vi "S8300E_Revision_Test_WIH.vi"() -> ()   [LabVIEW 2011]
panel:
  out "PRELOG2":string
  out "PRELOG1":string
  out "UUT_LAN_FW_VERSION":string
  out "CPK_SUFFIX":string
  out "Vintage_Number":string
  out "CPLD_Version":string
  out "Log":string
  out "MSG List":string[](array[string])
  out "VISA resource name out":refnum<visa-resource-name>
  out "Cmd Line":cluster{string, string, "BIST Version":string}[](array[cluster])
  out "BIST Version":string
  out "OS Version":string
  out "BIOS_VERSION":string
  out "BEGIN TIME":u32
  out "進行狀況":string
  # "Error Code:Version\nError Code:UART"
  # "2015-6-1"
  # "S8300E Version Check (接UART COM9)"
  # "Baud-Rate:115200"
  # "Step1:BIOS Version Check\nStep2:OS Version\nStep3:BIST\nStep4:Get CPLD device ID and revision number\nStep5:Get Vintage Number of the Circuit Pack\nStep6:Get Suffix of the Circuit Pack\nStep7:Get SuperIO Device ID\nStep8:Get Clock Generator ID\nStep9:Get LAN EEPROM firmware verson"
  # "Rule :bits [7-4] : CPLD Device ID, S8300E CPLD Device ID=4\nbits [3-0] : CPLD Revision Number"
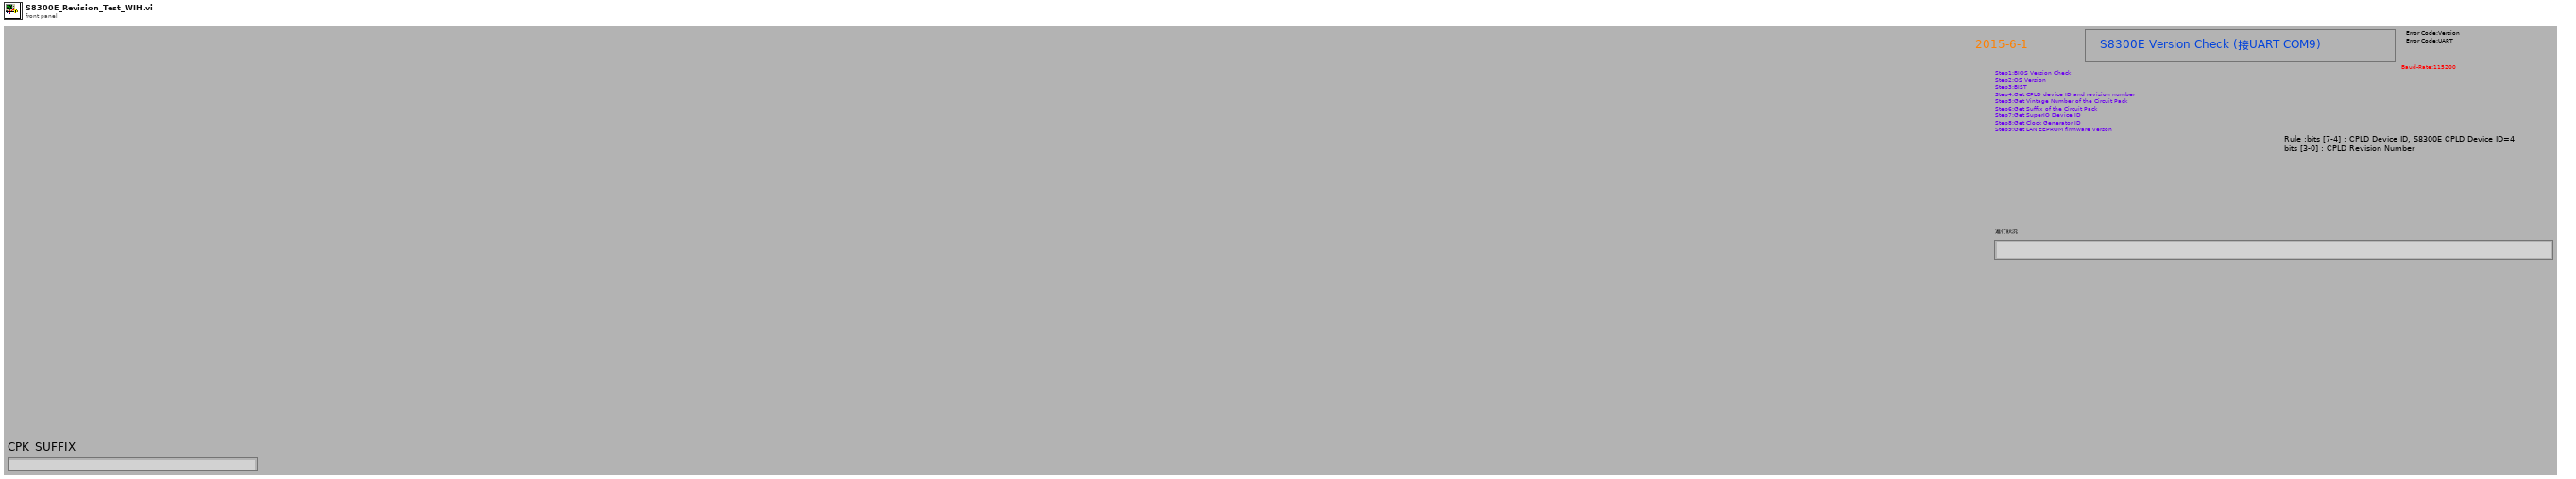
[diagram p1: front panel]
types:
  T1 = cluster{string, string, "UUT_LAN_FW_VERSION":string}
  T2 = cluster{string, string, "UUT_LAN_FW_VERSION":string}[]
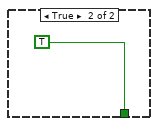
[diagram p5: hidden frame]
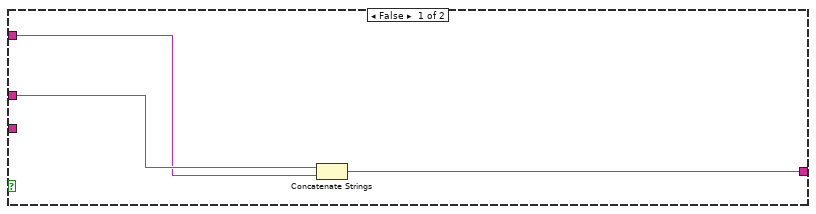
[diagram p6: hidden frame]
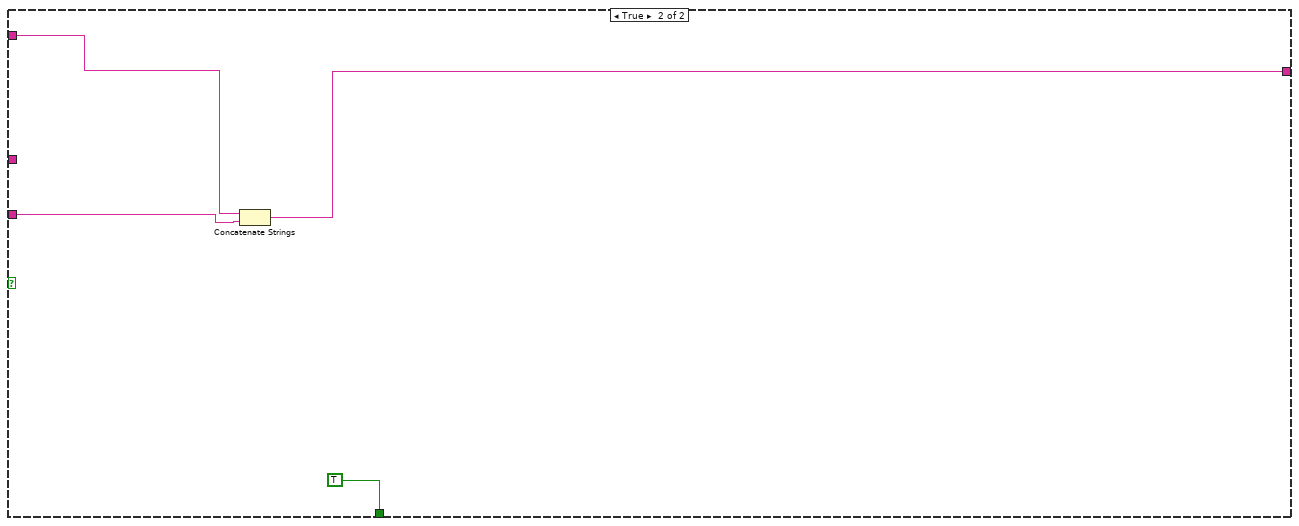
[diagram p7: hidden frame]
diagram:
  n1 = flat-sequence {
    frame #0 {
      n2 = Tick Count (ms)() -> (millisecond timer value=→"BEGIN TIME":u32)
    }
    frame #1 {
      n3 = property on="進行狀況" class="Str"("Blinking"=TRUE) -> ()  [unwired: 2 in, 2 out]
      "進行狀況" <- "進入測試準備中...." ("進行狀況")
    }
    frame #2 {
      n4 = call "SUB_SearchFile_inFolder.vi"("Search Filename in Folder"="S8300E_sfcs_misc.txt") -> ("File Existing True/Flase"=w4:bool)  [unwired: 1 in]
      n5 = case shown="False" w4 {
        frame False {
          n6 = flat-sequence {
            frame #0 {
              n7 = call "Display Message to User"() -> ()  [unwired: 10 in, 2 out]
            }
            frame #1 {
              n8 = call "SUB_Writelog.vi"("Pass/Fail"="Fail:S8300E_Revision_Test") -> ()  [unwired: 2 in]
            }
            frame #2 {
              n9 = Quit LabVIEW(quit? (T)=TRUE) -> ()
            }
          }
        }
        frame True {
        }
      }
    }
    frame #3 {
      n10 = call "SUB_ReadScript_File.vi"("Script FileName"="S8300E_sfcs_misc.txt" ("Search Filename in Folder")) -> ("text"=w12:string)  [unwired: 1 in, 2 out]
      n11 = call "SUB_FindSpecificString.vi"("Find this String"="UUT_CPLD_VERSION=", "String data"=w12) -> ("before \"; \" string"=→"CPLD_Version":string, "Found"=w17:bool)  [unwired: 2 in]
      n12 = call "SUB_FindSpecificString.vi"("Find this String"="UUT_OS_VERSION=", "String data"=w12) -> ("before \"; \" string"=→"OS Version":string, "Found"=w28:bool)  [unwired: 2 in]
      n13 = call "SUB_FindSpecificString.vi"("Find this String"="UUT_BIST_VERSION=", "String data"=w12) -> ("before \"; \" string"=→"BIST Version":string, "Found"=w26:bool)  [unwired: 2 in]
      n14 = call "SUB_FindSpecificString.vi"("Find this String"="UUT_VintageNumber=", "String data"=w12) -> ("before \"; \" string"=→"Vintage_Number":string, "Found"=w19:bool)  [unwired: 2 in]
      n15 = call "SUB_FindSpecificString.vi"("Find this String"="UUT_CircuitPack_SUFFIX=", "String data"=w12) -> ("before \"; \" string"=→"CPK_SUFFIX":string, "Found"=w18:bool)  [unwired: 2 in]
      n16 = call "SUB_FindSpecificString.vi"("Find this String"="UUT_BIOS_VERSION=", "String data"=w12) -> ("before \"; \" string"=→"BIOS_VERSION":string, "Found"=w29:bool)  [unwired: 2 in]
      n17 = call "SUB_FindSpecificString.vi"("Find this String"="UUT_LAN_FW_VERSION=", "String data"=w12) -> ("before \"; \" string"=→"UUT_LAN_FW_VERSION":string, "Found"=w10:bool)  [unwired: 2 in]
      n18 = And(x=w19, y=w18) -> (x .and. y?=w11:bool)
      n19 = And(x=w11, y=w10) -> (x .and. y?=w9:bool)
      n20 = And(x=w17, y=w9) -> (x .and. y?=w15:bool)
      n21 = And(x=w29, y=w28) -> (x .and. y?=w27:bool)
      n22 = And(x=w27, y=w26) -> (x .and. y?=w16:bool)
      n23 = And(x=w16, y=w15) -> (x .and. y?=w14:bool)
      n24 = case shown="False" w14 {
        frame False {
          n25 = flat-sequence {
            frame #0 {
              n26 = call "Display Message to User2"() -> ()  [unwired: 10 in, 2 out]
            }
            frame #1 {
              n27 = call "SUB_Writelog.vi"("Pass/Fail"="Fail:S8300E_Revision_Test") -> ()  [unwired: 2 in]
            }
            frame #2 {
              n28 = Quit LabVIEW(quit? (T)=TRUE) -> ()
            }
          }
        }
        frame True {
        }
      }
    }
    frame #4 {
      (unwired) "PASSED="
      (unwired) "PASSED="
      n29 = local read "BIST Version"() -> (w44:string)
      n30 = local read "OS Version"() -> (w48:string)
      n31 = local read "BIOS_VERSION"() -> (w53:string)
      n32 = local read "CPLD_Version"() -> (w83:string)
      n33 = local read "Vintage_Number"() -> (w80:string)
      n34 = local read "UUT_LAN_FW_VERSION"() -> (w40:string)
      n35 = local read "CPK_SUFFIX"() -> (w77:string)
      n36 = Concatenate Strings("PASSED=", w53, ";") -> (w51:string)
      n37 = Concatenate Strings("PASSED=", w48, ";") -> (w47:string)
      n38 = Concatenate Strings("PASSED=", w44, ";") -> (w43:string)
      n39 = Concatenate Strings("PASSED=", w40, ";") -> (w39:string)
      n40 = Bundle("./ver.sh -t", w43, "BIST Version"=w44) -> (w94:cluster{string, string, "BIST Version":string})  [unwired: 1 in]
      n41 = Bundle("./ver.sh -b", w51, "BIOS_VERSION"=w53) -> (w96:cluster{string, string, "BIOS_VERSION":string})  [unwired: 1 in]
      n42 = Bundle("./ver.sh -o", w47, "OS Version"=w48) -> (w95:cluster{string, string, "OS Version":string})  [unwired: 1 in]
      n43 = Bundle("./ver.sh -v", "PASSED=", "Vintage_Number"=w80) -> (w75:cluster{string, string, "Vintage_Number":string})  [unwired: 1 in]
      n44 = Bundle("./ver.sh -c", "PASSED=", "CPLD_Version"=w83) -> (w76:cluster{string, string, "CPLD_Version":string})  [unwired: 1 in]
      n45 = Bundle("./ver.sh -s", "PASSED=", "CPK_SUFFIX"=w77) -> (w74:cluster{string, string, "CPK_SUFFIX":string})  [unwired: 1 in]
      n46 = Bundle("./ver.sh -g", "PASSED=", "0X42") -> (w65:cluster{string, string, string})  [unwired: 1 in]
      n47 = Bundle("./eth.sh -f  1", w39, "UUT_LAN_FW_VERSION"=w40) -> (w60:T1)  [unwired: 1 in]
      n48 = Bundle("./eth.sh -f  2", w39, "UUT_LAN_FW_VERSION"=w40) -> (w59:T1)  [unwired: 1 in]
      n49 = Bundle("./ver.sh -p", "PASSED=", "Found IT8612F chip at 0xa20") -> (w70:cluster{string, string, string})  [unwired: 1 in]
      n50 = Bundle("./eth.sh -f   3", w39, "UUT_LAN_FW_VERSION"=w40) -> (w58:T1)  [unwired: 1 in]
      n51 = Build Array("正在處理BIOS版本中....", "正在處理OS版本中....", "正在處理BIST版本中....", "正在處理CPLD版本中....", "正在處理 Vintage Number of the Circuit Pack....", "正在處理Suffix of the Circuit Pack....", "正在處理SuperIO Device", "Get Clock Generator ID", "Get  LAN FW Version Port1", "Get  LAN FW Version Port2", "Get  LAN FW Version Port3") -> (→"MSG List":string[])
      n52 = Build Array(w96, w95, w94, w76, w75, w74, w70, w65, w60, w59, w58) -> (→"Cmd Line":T2)
    }
    frame #5 {
      n53 = call "SUB_COM1_CLOSE.vi"("VISA resource name"=refnum<visa-resource-name> "COM9") -> ()  [unwired: 3 in]
    }
    frame #6 {
      n54 = call "SUB_COM9_INIT.vi"("baud rate"=u32 115200) -> ("VISA resource name out"=w104:refnum<visa-resource-name>)  [unwired: 1 in, 1 out]
      "VISA resource name out" <- w104
      n55 = call "SUB_COM1Wrt.vi"("VISA resource name"=w104, "write buffer"="\r") -> ("duplicate VISA resource name"=w101:refnum<visa-resource-name>)  [unwired: 1 in, 1 out]
      n56 = call "SUB_ContinueCom1Read.vi"("Numeric"=1200, "duplicate VISA resource name 2"=w101) -> ()  [unwired: 1 in, 3 out]
    }
    frame #7 {
      n57 = while {
        stop <- w115 stop-if-true
        n58 = Tick Count (ms)() -> (millisecond timer value=w109:u32)
        n59 = local read "VISA resource name out"() -> (w107:refnum<visa-resource-name>)
        n60 = call "SUB_ContinueCom1Read.vi"("Numeric"=1200, "duplicate VISA resource name 2"=w107) -> ("duplicate VISA resource name"=w106:refnum<visa-resource-name>)  [unwired: 1 in, 2 out]
        n61 = call "SUB_COM1Wrt.vi"("VISA resource name"=w106, "write buffer"="\r") -> ("duplicate VISA resource name"=w111:refnum<visa-resource-name>)  [unwired: 1 in, 1 out]
        n62 = call "SUB_READ_COM1_FindString_timeout.vi"("Find this String"="S8300E", "Timeout Seccond"=2.0, "Begin time"=w109, "duplicate VISA resource name 2"=w111) -> ("Output String"=w112:string, "Found String"=w113:bool)  [unwired: 1 in, 1 out]
        n63 = case shown="False" w113 {
          tunnel: w112 -> [w121 _]
          tunnel: [w117 TRUE] -> w115
          frame False {
            n64 = call "SUB_YESNO.vi"("Debug View"=w121, "Status"="UART無正確反應!需有S8300E字串") -> ("yes/no"=w120:enum32{"No Selection", "Yes", "No", "None"})  [unwired: 1 in]
            n65 = Equal?(x=w120, y=enum32{"No Selection", "Yes", "No", "None"}."No") -> (x = y?=w118:bool)
            n66 = case shown="True" w118 {
              tunnel: [_ w123] -> w117
              frame False {
              }
              frame True {
                n67 = flat-sequence {
                  tunnel: [w127] -> w123
                  frame #0 {
                    n68 = call "SUB_Writelog.vi"("Pass/Fail"="Fail:S8300E_Revision_Test") -> ()  [unwired: 2 in]
                  }
                  frame #1 {
                    n69 = call "SUB_SFCS_SendResult.vi"("ErrorCode"="UART", "PASS_Fail (1/0)"=i8 0) -> ()  [unwired: 1 out]
                  }
                  frame #2 {
                    w127 = TRUE ("quit? (T)")
                    n70 = Quit LabVIEW(quit? (T)=w127) -> ()
                  }
                }
              }
            }
          }
          frame True {
          }
        }
      }
    }
    frame #8 {
      n71 = local read "Cmd Line"() -> (w132:cluster{string, string, "BIST Version":string}[])
      n72 = Array Size(array=w132) -> (size(s)=w131:i32)
      n73 = for {
        N: w131 -> [_]
        shift-right: [w135] -> w129
        shift-left: "" -> [w133]
        i -> [w137]
        n74 = while {
          tunnel: w137 -> [w162]
          shift-right: [w149] -> w136
          shift-left: "" -> [w147]
          stop <- w159 stop-if-true
          n75 = local read "VISA resource name out"() -> (w145:refnum<visa-resource-name>)
          n76 = local read "Cmd Line"() -> (w161:cluster{string, string, "BIST Version":string}[])
          n77 = Index Array(array=w161, index=w162) -> (element=w160:cluster{string, string, "BIST Version":string})
          n78 = call "SUB_ContinueCom1Read.vi"("Numeric"=1200, "duplicate VISA resource name 2"=w145) -> ("duplicate VISA resource name"=w144:refnum<visa-resource-name>)  [unwired: 1 in, 2 out]
          n79 = Unbundle(w160) -> (w158:string, w153:string, "BIST Version"=w152:string)
          n80 = Concatenate Strings(w158, "\r") -> (w143:string)
          n81 = call "SUB_COM1Wrt.vi"("VISA resource name"=w144, "write buffer"=w143) -> ("duplicate VISA resource name"=w156:refnum<visa-resource-name>)  [unwired: 1 in, 1 out]
          n82 = Tick Count (ms)() -> (millisecond timer value=w154:u32)
          n83 = To Upper Case(1:w152) -> (0:w151:string)
          n84 = call "SUB_READ_COM1_FindString_timeout.vi"("Find this String"=w153, "Timeout Seccond"=2.0, "Begin time"=w154, "duplicate VISA resource name 2"=w156) -> ("Output String"=w142:string)  [unwired: 1 in, 2 out]
          n85 = call "SUB_FindSpecificString.vi"("Find this String"=w153, "String data"=w142) -> ()  [unwired: 2 in, 2 out]
          n86 = call "SUB_FindSpecificString.vi"("Find this String"=w151, "String data"=w142) -> ("Found"=w150:bool)  [unwired: 2 in, 1 out]
          n87 = Concatenate Strings(w143, w142, "\n") -> (w140:string)
          n88 = case shown="False" w150 {
            tunnel: w142 -> [w166 w194]
            tunnel: [w163 w192] -> w148
            tunnel: [_ TRUE] -> w159
            tunnel: w151 -> [w167 _]
            tunnel: w140 -> [w164 w191]
            frame False {
              n89 = local read "進行狀況"() -> (w168:string)
              n90 = Concatenate Strings("Fail:Unmatch !版本與定義不符合! 系統需回" ("string"), w167, "\r", w168) -> (w165:string)
              n91 = call "SUB_YESNO.vi"("Debug View"=w166, "Status"=w165) -> ("yes/no"=w173:enum32{"No Selection", "Yes", "No", "None"})  [unwired: 1 in]
              n92 = Equal?(x=w173, y=enum32{"No Selection", "Yes", "No", "None"}."No") -> (x = y?=w170:bool)
              n93 = case shown="True" w170 {
                tunnel: w166 -> [_ w178]
                tunnel: w165 -> [w176 w177]
                tunnel: w164 -> [w175 _]
                tunnel: [w174 _] -> w163
                frame False {
                  n94 = Concatenate Strings(w176, w175) -> (w174:string)
                }
                frame True {
                  n95 = flat-sequence {
                    tunnel: w178 -> [w180]
                    tunnel: w177 -> [w182]
                    tunnel: [w190] -> _
                    frame #0 {
                      w183 = "\n"
                      n96 = local read "PRELOG2"() -> (w185:string)
                      n97 = local read "PRELOG1"() -> (w184:string)
                      n98 = Concatenate Strings(w182, "\n", w180) -> (w179:string)
                      n99 = Concatenate Strings("Fail:S8300E_Revision Test" ("Pass/Fail"), w183, w185, w183, w184, w183, w179) -> (w186:string)
                      n100 = call "SUB_Writelog.vi"("Pass/Fail"=w186) -> ()  [unwired: 2 in]
                    }
                    frame #1 {
                      n101 = call "SUB_SFCS_SendResult.vi"("ErrorCode"="Version", "PASS_Fail (1/0)"=i8 0) -> ()  [unwired: 1 out]
                    }
                    frame #2 {
                      w190 = TRUE ("quit? (T)")
                      n102 = Quit LabVIEW(quit? (T)=w190) -> ()
                    }
                  }
                }
              }
            }
            frame True {
              n103 = Concatenate Strings(w191, w194) -> (w192:string)
            }
          }
          n104 = Concatenate Strings(w147, w148) -> (w149:string)
          "PRELOG1" <- w149
        }
        n105 = local read "MSG List"() -> (w139:string[])
        n106 = Index Array(array=w139, index=w137) -> (element=w138:string)
        n107 = local write "進行狀況"(w138) -> ()
        n108 = Concatenate Strings(w133, w136) -> (w135:string)
        "PRELOG2" <- w135
      }
      "Log" <- w129
    }
    frame #9 {
      n109 = call "SUB_COM1_CLOSE.vi"("VISA resource name"=refnum<visa-resource-name> "COM9") -> ()  [unwired: 3 in]
    }
    frame #10 {
      w198 = "***Not Good ***" ("replace string (\"\")")
      n110 = local read "BEGIN TIME"() -> (w207:u32)
      n111 = Tick Count (ms)() -> (millisecond timer value=w206:u32)
      n112 = call "SUB_CAL_TESTTIME.vi"("Test Item name"="S8300E_Revision_Test", "Stop tick time"=w206, "Start tick time"=w207) -> ("Test Time output"=w202:string)  [unwired: 2 in]
      n113 = local read "Log"() -> (w203:string)
      n114 = Concatenate Strings("Pass:S8300E_Revision_Test", "\n", w203, w202) -> (w196:string)
      n115 = call "SUB_SEARCH_REPLACE_STR.vi"("replace string (\"\")"=w198, "search string"="FAILED", "input string"=w196) -> ("result string"=w200:string)  [unwired: 2 in]
      n116 = call "SUB_SEARCH_REPLACE_STR.vi"("replace string (\"\")"=w198, "search string"="FAIL", "input string"=w200) -> ("result string"=w197:string)  [unwired: 2 in]
      n117 = call "SUB_Writelog.vi"("Pass/Fail"=w197) -> ()  [unwired: 2 in]
    }
    frame #11 {
      n118 = Quit LabVIEW(quit? (T)=TRUE ("stop? (T)")) -> ()
    }
  }
